vi "AlliGator Get Complementary Channel Names.vi"(8 "Error In":errorcluster, 10 "Selected Channel Name":string, 11 "Available Channel Names":string[](array[string])) -> (0 "Error Out":errorcluster, 1 "G2 Channel Name (or single Gate Name)":string, 2 "Selected Channel Name (dup)":string, 3 "Complementary Channel Name (or empty)":string, 4 "INT Channel Name (or empty)":string, 5 "Dataset Channel":T1)   [LabVIEW 2021, in "AlliGator Files.lvlib"]
doc: "Obtains information on channel names from the <B>Selected Channel Name</B>."
uses:
  AlliGator Files.lvlib
  Dual-Channel Datasets/AlliGator Dataset Channel.ctl
  Dual-Channel Datasets/AlliGator Dual-Channel Datasets.lvlib
panel:
  # "see the AlliGator License on the block diagram (Ctrl+E or Window:Show Block Diagram)"
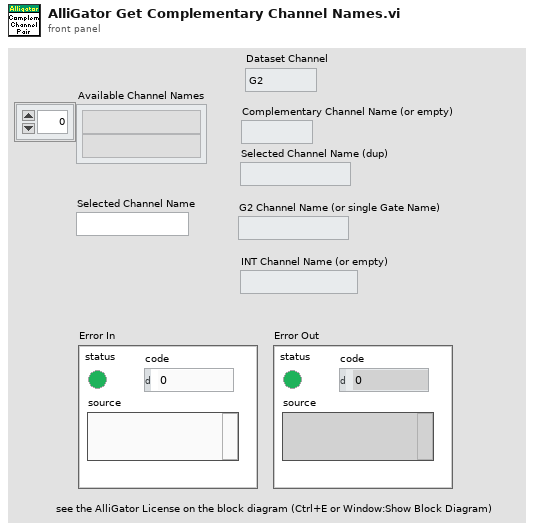
[diagram p1: front panel]
types:
  T1 = typedef "AlliGator Dual-Channel Datasets.lvlib/AlliGator Dataset Channel.ctl" = enum16{"G2", "INT"}
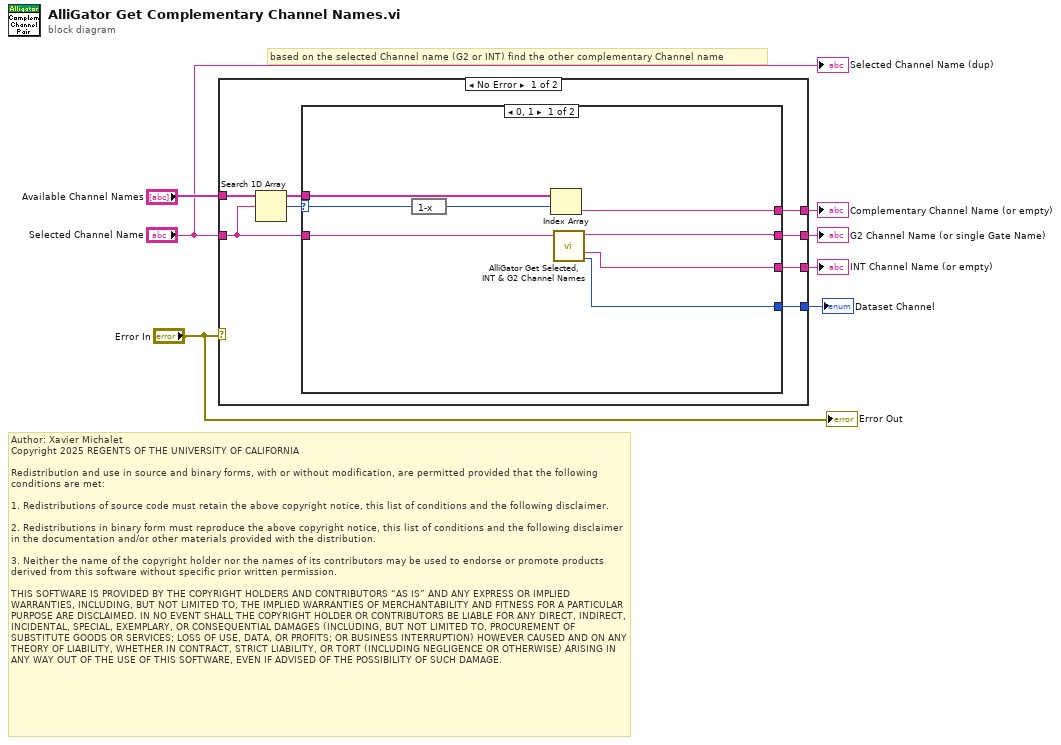
[diagram p0: block diagram]
diagram:
  # "Author: Xavier Michalet\nCopyright 2025 REGENTS OF THE UNIVERSITY OF CALIFORNIA\n\nRedistribution and use in source and binary forms, with or without modification, are permitted provided that the following conditions are met:\n\n1. Redistributions of source code must retain the above copyright notice, this list of conditions and the following disclaimer.\n\n2. Redistributions in binary form must reproduce the above copyright notice, this list of conditions and the following disclaimer in the documentation and/or other materials provided with the distribution.\n\n3. Neither the name of the copyright holder nor the names of its contributors may be used to endorse or promote products derived from this software without specific prior written permission.\n\nTHIS SOFTWARE IS PROVIDED BY THE COPYRIGHT HOLDERS AND CONTRIBUTORS “AS IS” AND ANY EXPRESS OR IMPLIED WARRANTIES, INCLUDING, BUT NOT LIMITED TO, THE IMPLIED WARRANTIES OF MERCHANTABILITY AND FITNESS FOR A PARTICULAR PURPOSE ARE DISCLAIMED. IN NO EVENT SHALL THE COPYRIGHT HOLDER OR CONTRIBUTORS BE LIABLE FOR ANY DIRECT, INDIRECT, INCIDENTAL, SPECIAL, EXEMPLARY, OR CONSEQUENTIAL DAMAGES (INCLUDING, BUT NOT LIMITED TO, PROCUREMENT OF SUBSTITUTE GOODS OR SERVICES; LOSS OF USE, DATA, OR PROFITS; OR BUSINESS INTERRUPTION) HOWEVER CAUSED AND ON ANY THEORY OF LIABILITY, WHETHER IN CONTRACT, STRICT LIABILITY, OR TORT (INCLUDING NEGLIGENCE OR OTHERWISE) ARISING IN ANY WAY OUT OF THE USE OF THIS SOFTWARE, EVEN IF ADVISED OF THE POSSIBILITY OF SUCH DAMAGE."
  # "based on the selected Channel name (G2 or INT) find the other complementary Channel name"
  n1 = case shown="No Error" "Error In" {
    tunnel: "Available Channel Names" -> [w10 _]
    tunnel: "Selected Channel Name" -> [w13 w24]
    tunnel: [w12 w24] -> w3
    tunnel: [w11 _] -> w6
    tunnel: [w9 _] -> w2
    tunnel: [w8 _] -> w1
    frame No Error {
      n2 = Search 1D Array(1D array=w10, element=w13) -> (index of element=w14:i32)  [unwired: 1 in]
      n3 = case shown="0, 1" w14 {
        selector: w14 -> [w18 _]
        tunnel: w13 -> [w22 w23]
        tunnel: [w21 w23] -> w12
        tunnel: [w20 _] -> w11
        tunnel: w10 -> [w19 _]
        tunnel: [w16 _] -> w9
        tunnel: [w15 _] -> w8
        frame 0, 1 {
          n4 = expression code="1-x"(w18) -> (w17:i32)
          n5 = Index Array(array=w19, index=w17) -> (element=w16:string)
          n6 = call "AlliGator Get Selected, INT & G2 Channel Names.vi"("Selected Channel Name in"=w22) -> ("Dataset Channel"=w15:T1, "INT Channel Name (or empty)"=w20:string, "G2 Channel Name (or single Channel Name)"=w21:string)  [unwired: 8 in]
        }
        frame ..-1, Default {
          # "Not found'"
        }
      }
    }
    frame Error {
    }
  }
  "INT Channel Name (or empty)" <- w6
  "G2 Channel Name (or single Gate Name)" <- w3
  "Complementary Channel Name (or empty)" <- w2
  "Dataset Channel" <- w1
  "Selected Channel Name (dup)" <- "Selected Channel Name"
  "Error Out" <- "Error In"
